vi "GSIOC buffered.vi"(8 "error in (no error)":errorcluster, 10 "Bufferd command":string, 11 "VISA resource name":refnum<visa-resource-name>="COM1") -> (0 "error out":errorcluster, 2 "Device busy":bool, 3 "VISA resource name out":refnum<visa-resource-name>)   [LabVIEW 2015]
panel:
  out "Array":string[](array[string])
  out "read buffer":string
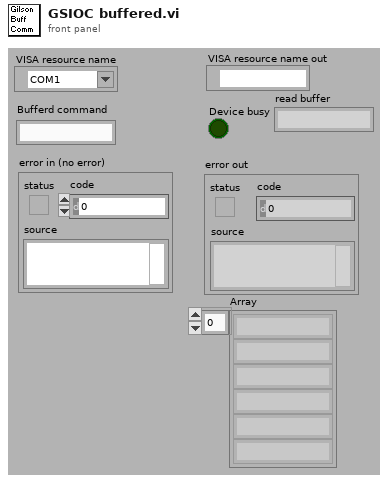
[diagram p1: front panel]
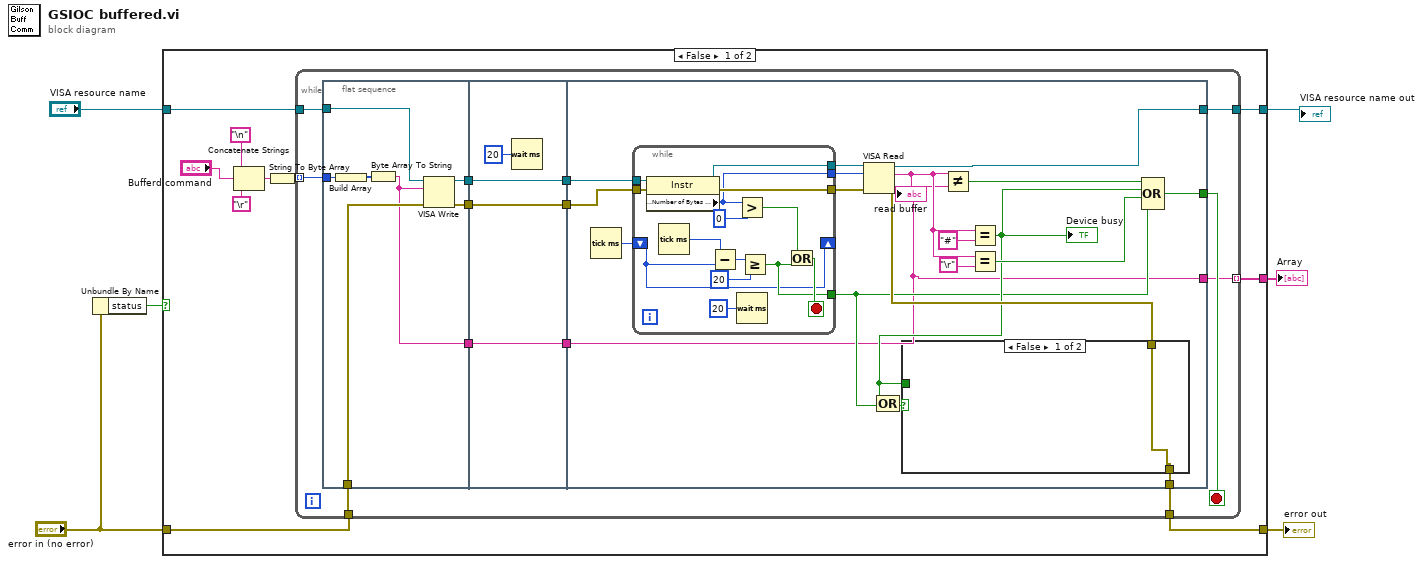
[diagram p0: block diagram]
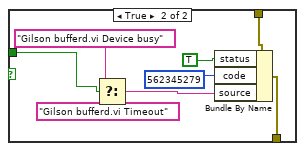
[diagram p2: hidden frame]
diagram:
  n1 = Unbundle By Name("error in (no error)") -> ("status"=w5:bool)
  n2 = case shown="False" w5 {
    tunnel: "error in (no error)" -> [w16 w84]
    tunnel: [w10 w84] -> w4
    tunnel: "VISA resource name" -> [w9 w83]
    tunnel: [w8 w83] -> w2
    tunnel: [w7 _] -> w1
    frame False {
      n3 = Concatenate Strings("\n", "Bufferd command", "\r") -> (w15:string)
      n4 = String To Byte Array(string=w15) -> (unsigned byte array=w11:u8[])
      n5 = while {
        tunnel: w16 -> [w23]
        tunnel: w11 -> [w22] mode=indexing
        tunnel: [w21] -> w10
        tunnel: w9 -> [w19]
        tunnel: [w18] -> w8
        tunnel: [w17] -> w7 mode=indexing
        stop <- w20 stop-if-true
        n6 = flat-sequence {
          tunnel: w23 -> [w36]
          tunnel: [w35] -> w29
          tunnel: [w34] -> w28
          tunnel: [w31] -> w27
          tunnel: w22 -> [w33]
          tunnel: w19 -> [w30]
          tunnel: w29 -> [w40]
          tunnel: w28 -> [w39]
          tunnel: [w40] -> w26
          tunnel: [w39] -> w25
          tunnel: [w37] -> w24
          tunnel: w27 -> [w37]
          tunnel: w26 -> [w51]
          tunnel: w25 -> [w49]
          tunnel: w24 -> [w41]
          tunnel: [w47] -> w21
          tunnel: [w54] -> w20
          tunnel: [w42] -> w18
          tunnel: [w41] -> w17
          frame #0 {
            n7 = Build Array(w33) -> (w32:u8[])
            n8 = Byte Array To String(unsigned byte array=w32) -> (string=w31:string)
            n9 = VISA Write(VISA resource name=w30, write buffer=w31, error in (no error)=w36) -> (VISA resource name out=w35:refnum<visa-resource-name>, error out=w34:errorcluster)  [unwired: 1 out]
          }
          frame #1 {
            n10 = Wait (ms)(milliseconds to wait=u32 20) -> ()  [unwired: 1 out]
          }
          frame #2 {
            n11 = Tick Count (ms)() -> (millisecond timer value=w43:u32)
            n12 = while {
              tunnel: [w82] -> w52
              tunnel: w49 -> [w81]
              tunnel: w51 -> [w80]
              tunnel: [w79] -> w53
              tunnel: [w75] -> w50
              tunnel: [w70] -> w44
              shift-right: [w69] -> _
              shift-left: w43 -> [w69]
              stop <- w71 stop-if-true
              n13 = property class="Instr"(reference=w80, error in=w81) -> (reference out=w79:refnum<visa-resource-name>, error out=w82:errorcluster, "Serial Settings:Number of Bytes at Serial Port"=w75:u32)
              n14 = Tick Count (ms)() -> (millisecond timer value=w76:u32)
              n15 = Subtract(x=w76, y=w69) -> (x-y=w78:u32)
              n16 = Greater?(x=w75, y=u32 0) -> (0:w72:bool)
              n17 = Wait (ms)(milliseconds to wait=u32 20) -> ()  [unwired: 1 out]
              n18 = Greater Or Equal?(x=w78, y=u32 20) -> (x >= y?=w70:bool)
              n19 = Or(x=w72, y=w70) -> (x .or. y?=w71:bool)
            }
            n20 = VISA Read(VISA resource name=w53, byte count=w50, error in (no error)=w52) -> (VISA resource name out=w42:refnum<visa-resource-name>, read buffer=w55:string, error out=w48:errorcluster)  [unwired: 1 out]
            "read buffer" <- w55
            n21 = Not Equal?(x=w55, y=w41) -> (x != y?=w58:bool)
            n22 = Equal?(x=w55, y="#") -> (x = y?=w45:bool)
            "Device busy" <- w45
            n23 = Compound Arithmetic op=OR(w45, w44) -> (w46:bool)
            n24 = case shown="False" w46 {
              tunnel: w48 -> [w60 w68]
              tunnel: [w60 w67] -> w47
              tunnel: w45 -> [_ w63]
              frame False {
              }
              frame True {
                n25 = Select(t="Gilson bufferd.vi Device busy" ("source"), s=w63, f="Gilson bufferd.vi Timeout" ("source")) -> (s? t:f=w64:string)
                n26 = Bundle By Name(cluster=w68, "status"=TRUE, "code"=562345279, "source"=w64) -> (w67:errorcluster)
              }
            }
            n27 = Equal?(x=w55, y="\r") -> (x = y?=w56:bool)
            n28 = Compound Arithmetic op=OR(w58, w45, w56, w44) -> (w54:bool)
          }
        }
      }
    }
    frame True {
    }
  }
  "error out" <- w4
  "VISA resource name out" <- w2
  "Array" <- w1
